vi "Print.vi"(8 "Error In":errorcluster, 11 "reference in":refnum<class "MenuComponent.lvclass">) -> (0 "Error Out":errorcluster, 3 "reference out":refnum<class "MenuComponent.lvclass">)   [LabVIEW 2020, in "MenuComponent.lvclass"]
uses:
  MenuComponent.lvclass
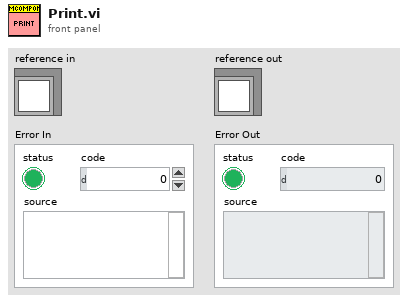
[diagram p1: front panel]
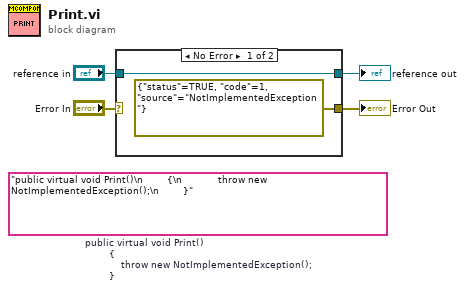
[diagram p0: block diagram]
diagram:
  (unwired) "public virtual void Print()\n        {\n            throw new NotImplementedException();\n        }"  # public virtual void Print()         {             throw new NotImplementedException();         }
  n1 = case shown="No Error" "Error In" {
    selector: "Error In" -> [_ w8]
    tunnel: [errorcluster {"status"=TRUE, "code"=1, "source"="NotImplementedException  "} ("error IO") w8] -> w3
    tunnel: [w5 w7] -> w1
    tunnel: "reference in" -> [w5 w7]
    frame No Error {
    }
    frame Error {
    }
  }
  "Error Out" <- w3
  "reference out" <- w1
